vi "Router - Writer.vi"(8 "error in (no error)":errorcluster, 9 "Reading Segments Array":T1[](array[typedef]), 10 "PXImc Writing Session In":refnum<k21>, 11 "Master Table Ref In":refnum<data-value>) -> (0 "error out":errorcluster)   [LabVIEW 2016, in "PXImc Router.lvlib"]
uses:
  PXImc Router.lvlib
  Controls/Table Index-Size.ctl
  <vilib>/pximc/Acquire Write Region (DBL).vi
  <vilib>/pximc/nipximc.lvlib
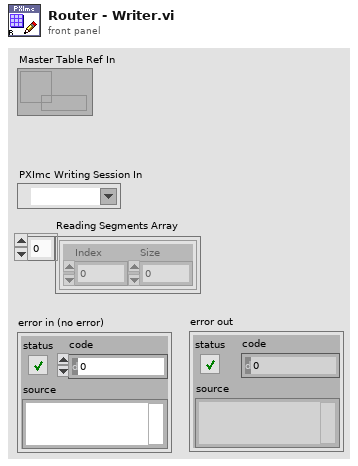
[diagram p1: front panel]
types:
  T1 = typedef "PXImc Router.lvlib/Table Index-Size.ctl" = cluster{"Index":u32, "Size":u32}
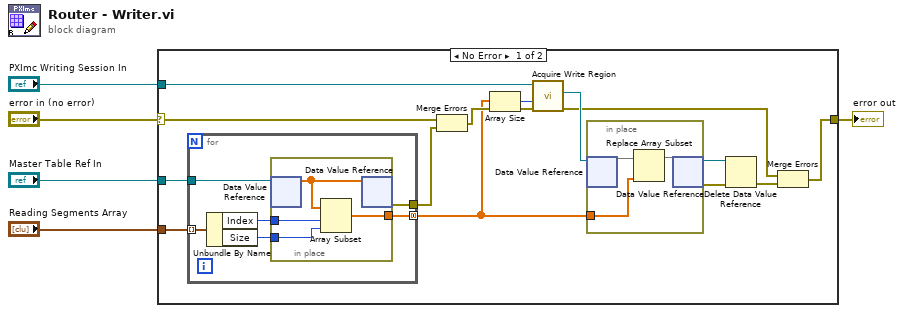
[diagram p0: block diagram]
diagram:
  n1 = case shown="No Error" "error in (no error)" {
    selector: "error in (no error)" -> [w16 w33]
    tunnel: "PXImc Writing Session In" -> [w19 _]
    tunnel: "Master Table Ref In" -> [w18 _]
    tunnel: [w17 w33] -> w4
    tunnel: "Reading Segments Array" -> [w15 _]
    frame No Error {
      n2 = for {
        tunnel: w18 -> [w25]
        tunnel: w15 -> [w24] mode=indexing
        tunnel: [w23] -> w8
        tunnel: [w20] -> w6 mode=concatenating
        n3 = Unbundle By Name(w24) -> ("Index"=w22:u32, "Size"=w21:u32)
        n4 = in-place {
          in-place-border: [w28] -> w20
          in-place-border: w22 -> [w27]
          in-place-border: w21 -> [w29]
          n5 = in-place-dvr #1(w25) -> (w26:dbl[])  [unwired: 1 out]
          n6 = Array Subset(array=w26, index=w27, length=w29) -> (w28:dbl[])
          n7 = in-place-dvr #1(w26) -> (w23:errorcluster)  [unwired: 1 out]
        }
      }
      n8 = Merge Errors(w16, w8) -> (w7:errorcluster)
      n9 = Array Size(array=w6) -> (size(s)=w9:i32)
      n10 = call-poly <vilib>:"Acquire Write Region.vi"("error in (no error)"=w7, "number of elements"=w9, "session in"=w19) -> ("error out"=w10:errorcluster, "write region reference"=w11:refnum<data-value>)  [unwired: 5 in, 2 out]
      n11 = in-place {
        in-place-border: w6 -> [w30]
        n12 = in-place-dvr #2(w11) -> (w32:dbl[])  [unwired: 1 out]
        n13 = Replace Array Subset(array=w32, new element=w30) -> (w31:dbl[])  [unwired: 1 in]
        n14 = in-place-dvr #2(w31) -> (w12:refnum<data-value>, w14:errorcluster)
      }
      n15 = Delete Data Value Reference(data value reference=w12, error in=w14) -> (error out=w13:errorcluster)  [unwired: 1 out]
      n16 = Merge Errors(w10, w13) -> (w17:errorcluster)
    }
    frame Error {
    }
  }
  "error out" <- w4
